vi "f_2_Qgc.vi"(0 "file path (IN)":path, 1 "Project #":string, 2 "Request #":string, 3 "TEST #":string, 5 "error in (no error)":errorcluster, 6 "VGE (-ve)":dbl, 8 "VGE (+ve)":dbl) -> (11 "Di (A)":dbl, 13 "Dt (ns)":dbl, 14 "file path (OUT)":path, 15 "Qgc - Delta Time (us)":dbl, 16 "Di/Dt (A/us)":dbl, 17 "DONE Qgc":bool, 18 "DONE Di/Dt ON":bool, 19 "error out":errorcluster)   [LabVIEW 2020]
uses:
  Global 1.vi
  <vilib>/measure/mamon.llb/Trigger Detection for 1 Channel.vi
  <vilib>/Analysis/NI_AALBase.lvlib
  <vilib>/measure/NI_MAPro.lvlib
panel:
  out "VGE <POINT B>":dbl
  out "Find Major in Histogram":dbl
  out "Histogram":dynamicdata(graph)
  out "Focus graph":waveform(dbl)(graph)
  in  "Decision ?":bool
  out "Dt (us)":dbl
  out "VGE constant point in Median Filter":dbl
  out "VGE <POINT A>":dbl
  out "Cursor c : Channel 2":dbl
  out "Cursor b : Channel 2":dbl
  out "Waveform Graph":waveform(dbl)[](graph)
  out "ON Region":waveform(dbl)[](graph) caption="Qgc"
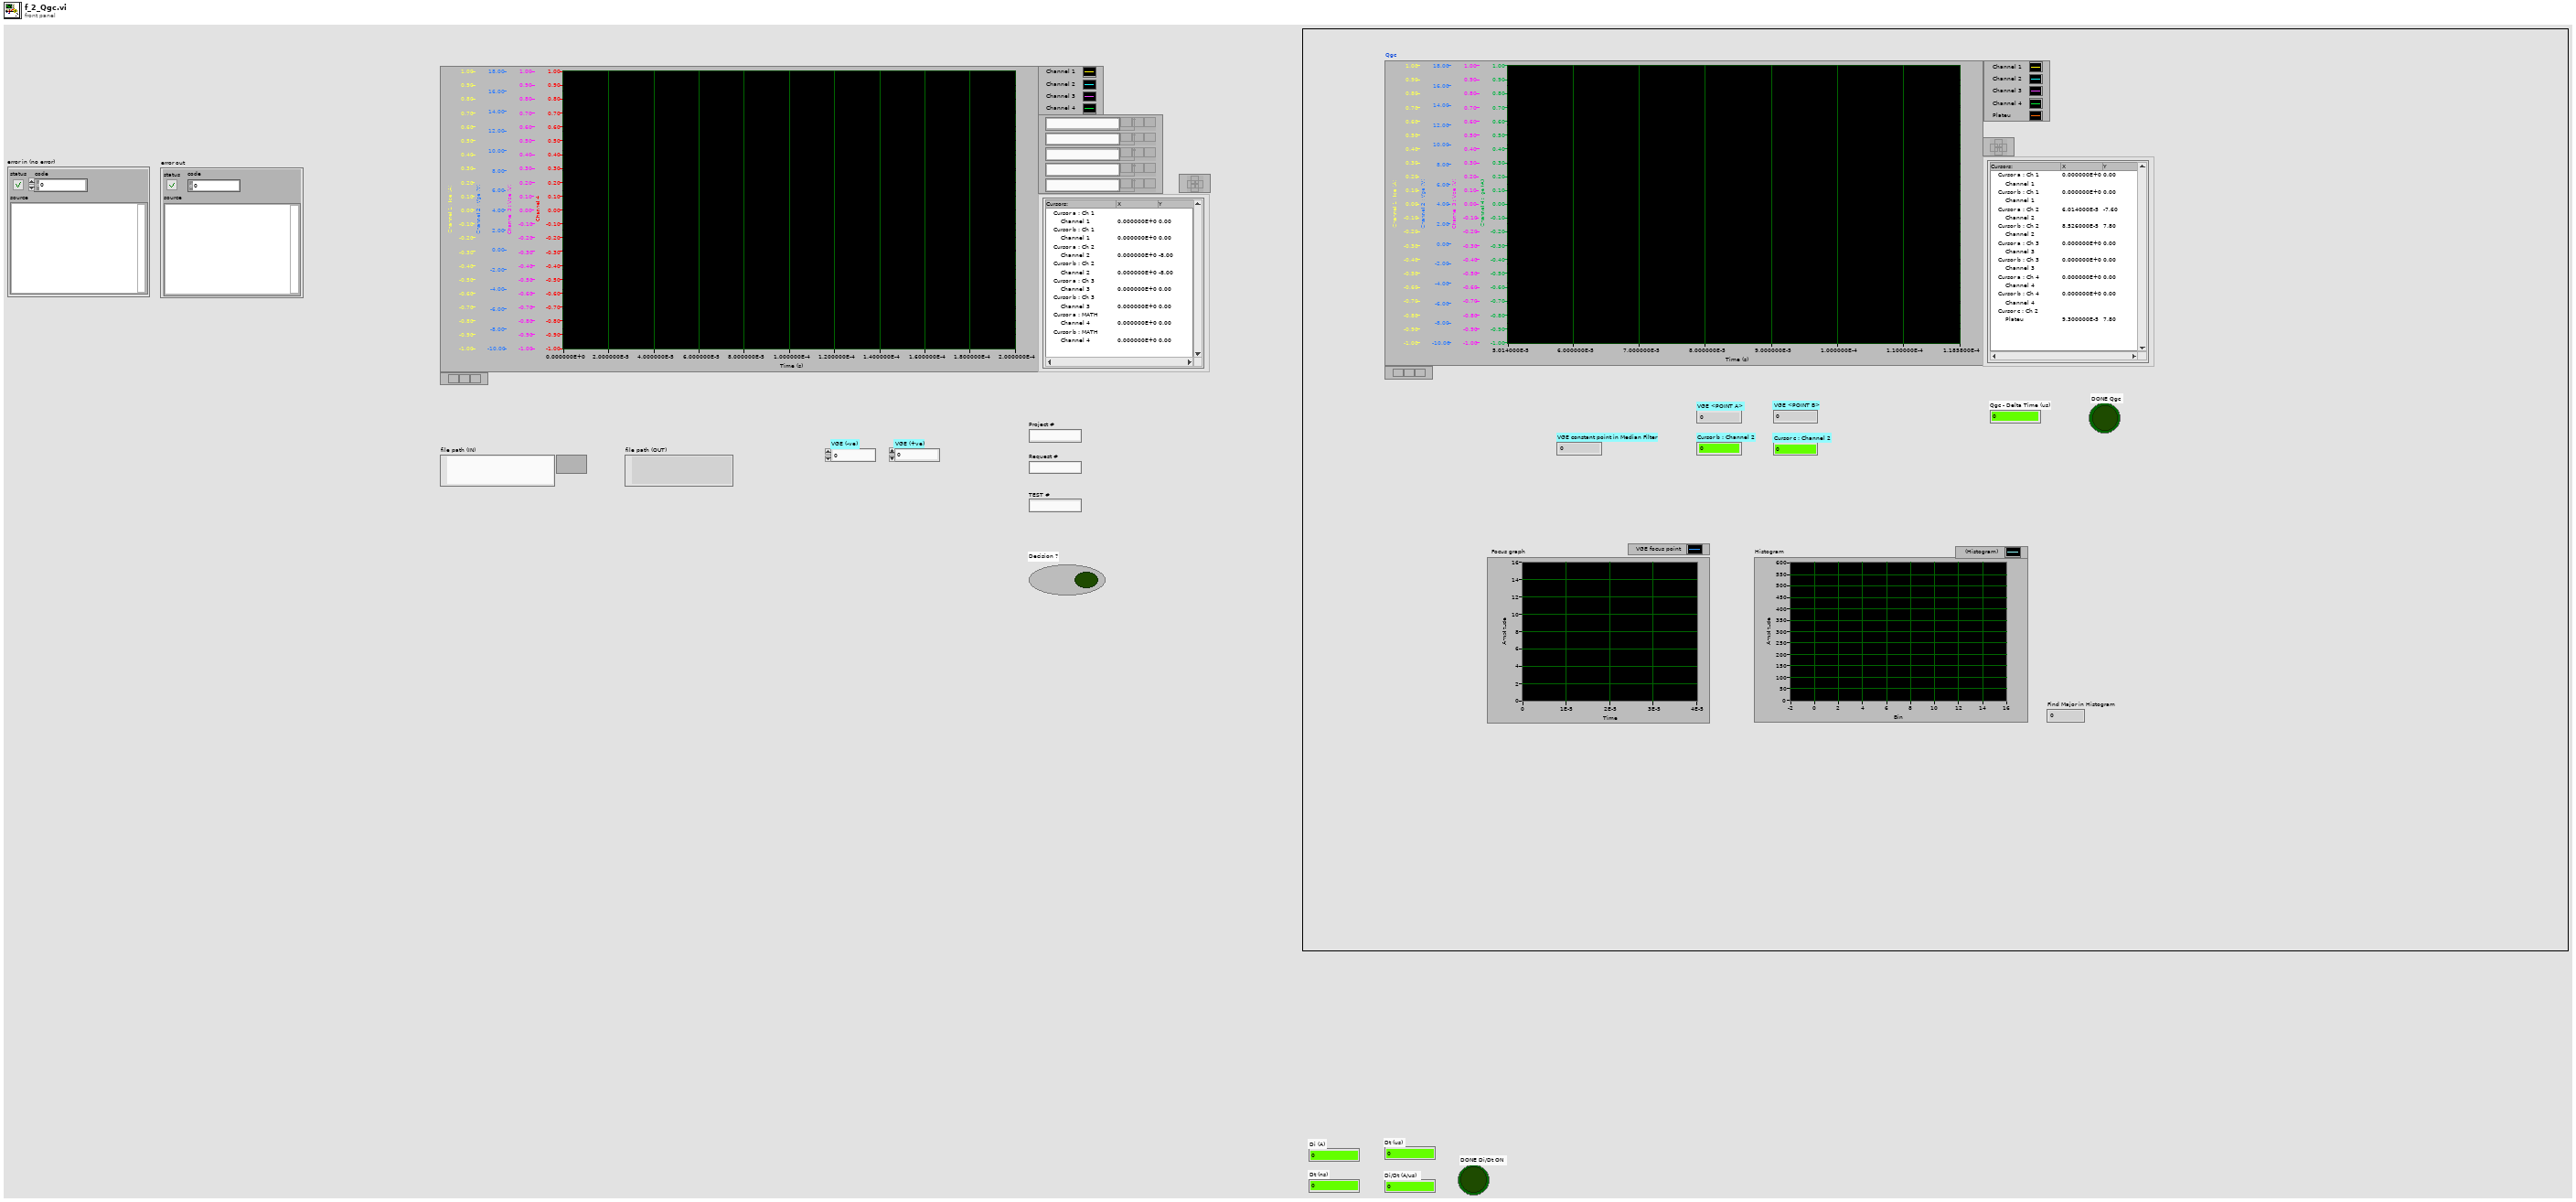
[diagram p1: front panel]
types:
  T1 = enum32{"Invalid", "Standard", "Closed", "Hidden", "Minimized", "Maximized"}
  T2 = typedef "imagedata.ctl" = cluster{"image type":i32, "image depth":i32, "image":u8[], "mask":u8[], "colors":u32[], "Rectangle":cluster{"left":i16, "top":i16, "right":i16, "bottom":i16}}
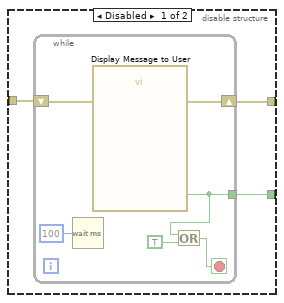
[diagram p2: hidden frame]
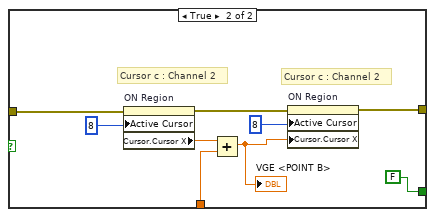
[diagram p9: hidden frame]
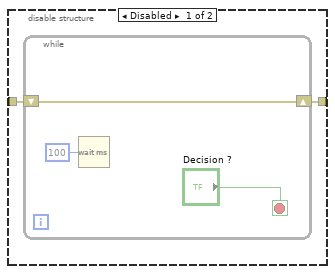
[diagram p11: hidden frame]
diagram:
  w5 = FALSE ("DONE Tdon")
  w1 = 0.0 ("Cursor a : Channel 1")
  w6 = errorcluster {"status"=FALSE, "code"=0, "source"=""} ("error out")
  w7 = waveform(dbl)[] [] ("Waveform Graph")
  n1 = local write "VGE constant point in Median Filter"(w1) -> ()
  n2 = local write "Qgc - Delta Time (us)"(w1) -> ()
  n3 = local write "DONE Qgc"(w5) -> ()
  n4 = local write "Cursor c : Channel 2"(w1) -> ()
  n5 = local write "Cursor b : Channel 2"(w1) -> ()
  n6 = local write "VGE <POINT A>"(w1) -> ()
  n7 = local write "VGE <POINT B>"(w1) -> ()
  n8 = local write "DONE Di/Dt ON"(w5) -> ()
  n9 = local write "Decision ?"(w5) -> ()
  n10 = local write "Di/Dt (A/us)"(w1) -> ()
  n11 = local write "Find Major in Histogram"(0.0 ("Time of Maximum")) -> ()
  n12 = local write "Di (A)"(w1) -> ()
  n13 = local write "Dt (ns)"(w1) -> ()
  n14 = local write "Dt (us)"(w1) -> ()
  n15 = local write "error out"(w6) -> ()
  n16 = local write "error in (no error)"(w6) -> ()
  n17 = local write "Waveform Graph"(w7) -> ()
  n18 = local write "ON Region"(w7) -> ()
  n19 = local write "Histogram"(dynamicdata [] ("Histogram")) -> ()
  n20 = local write "Focus graph"(waveform(dbl) {"t0"=timestamp(0 s since 1904-01-01), "dt"=1.0, "Y"=[]} ("Focus graph")) -> ()
  n21 = flat-sequence {
    tunnel: ["file path (IN)"] -> w13
    tunnel: [w14] -> w12
    tunnel: [w23] -> w11
    tunnel: [w22] -> w10
    tunnel: w13 -> [w25]
    tunnel: w12 -> [w24]
    tunnel: [w402] -> w9
    tunnel: w11 -> [w401]
    tunnel: w10 -> [w400]
    tunnel: [w400] -> w8
    tunnel: w9 -> [w417]
    tunnel: w8 -> [w416]
    frame #0 {
      n22 = control-ref of="This VI"() -> (w19:refnum<vi>)
      n23 = invoke class="VI" method="FP.Open"(reference=w19, error in="error in (no error)", "Activate"=TRUE ("Activate?"), "State"=T1."Maximized") -> (error out=w20:errorcluster)  [unwired: 1 in, 4 out]
      n24 = property class="VI"(reference=w19, error in=w20, "Front Panel.Closeable"=TRUE ("Front Panel Window:Closeable")) -> (error out=w14:errorcluster)  [unwired: 1 out]
    }
    frame #1 {
      n25 = while {
        tunnel: w25 -> [w85]
        shift-right: [w80] -> w23
        shift-left: w24 -> [w84]
        tunnel: [w82] -> w22
        stop <- w79 stop-if-true
        n26 = flat-sequence {
          tunnel: [w113] -> w94
          tunnel: [w114] -> w93
          tunnel: w85 -> [w114]
          tunnel: w84 -> [w113]
          tunnel: w94 -> [w132]
          tunnel: w93 -> [w130]
          tunnel: [w129] -> w75
          tunnel: [w121] -> w74
          tunnel: [w115] -> w73
          tunnel: [w116] -> w72
          tunnel: [w117] -> w71
          tunnel: [w119] -> w70
          tunnel: [w116] -> w46
          tunnel: w75 -> [w173]
          tunnel: [w173] -> w69
          tunnel: w74 -> [w172]
          tunnel: [w172] -> w67
          tunnel: w73 -> [w164]
          tunnel: w72 -> [w171]
          tunnel: w71 -> [w170]
          tunnel: [w170] -> w68
          tunnel: w70 -> [w169]
          tunnel: [w162] -> w66
          tunnel: w46 -> [w161]
          tunnel: [w161] -> w45
          tunnel: [w187] -> w78
          tunnel: w69 -> [w244]
          tunnel: [w244] -> w77
          tunnel: w68 -> [w243]
          tunnel: [w243] -> w76
          tunnel: w67 -> [w200]
          tunnel: w66 -> [w193]
          tunnel: w45 -> [w185]
          tunnel: [w185] -> w44
          tunnel: w78 -> [w258]
          tunnel: [w265] -> w58
          tunnel: w77 -> [w271]
          tunnel: [w271] -> w57
          tunnel: [w264] -> w56
          tunnel: [w245] -> w55
          tunnel: [w259] -> w54
          tunnel: w76 -> [w248]
          tunnel: [w248] -> w53
          tunnel: w44 -> [w247]
          tunnel: [w247] -> w43
          tunnel: w58 -> [w277]
          tunnel: [w284] -> w52
          tunnel: w57 -> [w291]
          tunnel: [w291] -> w51
          tunnel: w56 -> [w290]
          tunnel: [w290] -> w50
          tunnel: w55 -> [w283]
          tunnel: [w283] -> w49
          tunnel: w54 -> [w289]
          tunnel: [w289] -> w48
          tunnel: w53 -> [w288]
          tunnel: [w288] -> w47
          tunnel: w43 -> [w281]
          tunnel: [w281] -> w42
          tunnel: w52 -> [w294]
          tunnel: [w292] -> w41
          tunnel: w51 -> [w299]
          tunnel: [w299] -> w39
          tunnel: w50 -> [w298]
          tunnel: [w298] -> w36
          tunnel: w49 -> [w297]
          tunnel: [w297] -> w34
          tunnel: w48 -> [w296]
          tunnel: [w296] -> w32
          tunnel: w47 -> [w295]
          tunnel: [w295] -> w30
          tunnel: w42 -> [w293]
          tunnel: w41 -> [w331]
          tunnel: [w330] -> w40
          tunnel: w39 -> [w338]
          tunnel: [w338] -> w38
          tunnel: [w329] -> w37
          tunnel: w36 -> [w337]
          tunnel: [w337] -> w35
          tunnel: w34 -> [w336]
          tunnel: [w336] -> w33
          tunnel: w32 -> [w335]
          tunnel: [w335] -> w31
          tunnel: w30 -> [w334]
          tunnel: [w334] -> w29
          tunnel: [w328] -> w26
          tunnel: w40 -> [w344]
          tunnel: w38 -> [w352]
          tunnel: [w352] -> w65
          tunnel: w37 -> [w351]
          tunnel: [w351] -> w64
          tunnel: w35 -> [w350]
          tunnel: [w350] -> w63
          tunnel: w33 -> [w349]
          tunnel: [w349] -> w62
          tunnel: w31 -> [w348]
          tunnel: [w348] -> w61
          tunnel: [w343] -> w60
          tunnel: [w342] -> w59
          tunnel: w29 -> [w340]
          tunnel: [w339] -> w27
          tunnel: w26 -> [w339]
          tunnel: [w356] -> w92
          tunnel: w65 -> [w362]
          tunnel: [w362] -> w91
          tunnel: w64 -> [w361]
          tunnel: [w361] -> w90
          tunnel: w63 -> [w360]
          tunnel: [w360] -> w89
          tunnel: w62 -> [w358]
          tunnel: [w358] -> w88
          tunnel: w61 -> [w359]
          tunnel: w60 -> [w357]
          tunnel: w59 -> [w355]
          tunnel: [w353] -> w28
          tunnel: w27 -> [w353]
          tunnel: w92 -> [w375]
          tunnel: w91 -> [w386]
          tunnel: [w386] -> w87
          tunnel: w90 -> [w381]
          tunnel: w89 -> [w382]
          tunnel: w88 -> [w380]
          tunnel: [w375] -> w86
          tunnel: w28 -> [w373]
          tunnel: w87 -> [w391]
          tunnel: w86 -> [w393]
          tunnel: [w392] -> w81
          tunnel: [w391] -> w82
          frame #0 {
            w110 = waveform(dbl)[] [] ("Waveform Graph")
            w106 = 0.0 ("Cursor a : Channel 1")
            w112 = FALSE ("DONE Tdon")
            n27 = local write "VGE constant point in Median Filter"(w106) -> ()
            n28 = local write "Qgc - Delta Time (us)"(w106) -> ()
            n29 = local write "DONE Qgc"(w112) -> ()
            n30 = local write "Cursor c : Channel 2"(w106) -> ()
            n31 = local write "Cursor b : Channel 2"(w106) -> ()
            n32 = local write "VGE <POINT B>"(w106) -> ()
            n33 = local write "DONE Di/Dt ON"(w112) -> ()
            n34 = local write "Decision ?"(w112) -> ()
            n35 = local write "Di (A)"(w106) -> ()
            n36 = local write "Dt (ns)"(w106) -> ()
            n37 = local write "Dt (us)"(w106) -> ()
            n38 = local write "Di/Dt (A/us)"(w106) -> ()
            n39 = local write "VGE <POINT A>"(w106) -> ()
            n40 = Wait (ms)(milliseconds to wait=u32 200) -> ()  [unwired: 1 out]
            n41 = local write "Find Major in Histogram"(0.0 ("Time of Maximum")) -> ()
            n42 = local write "Histogram"(dynamicdata [] ("Histogram")) -> ()
            n43 = local write "ON Region"(w110) -> ()
            n44 = local write "Waveform Graph"(w110) -> ()
            n45 = local write "Focus graph"(waveform(dbl) {"t0"=timestamp(0 s since 1904-01-01), "dt"=1.0, "Y"=[]} ("Focus graph")) -> ()
          }
          frame #1 {
            w121 = 0.0 ("number")
            # "Channel 2"
            # "Channel 4"
            # "t0"
            # "Channel 1"
            # "Channel 3"
            # "dt"
            # "Ch1"
            n46 = call "3_ReadDatatoWaveform.vi"("file path (IN)"=w130, "error in (no error)"=w132) -> ("Ch 1 Data"=w128:dbl[], "Ch 2 Data"=w123:dbl[], "file path (OUT)"=w129:path, "Waveform Graph"=→"Waveform Graph":waveform(dbl)[], "Ch 3 Data"=w127:dbl[], "Ch 4 Data"=w125:dbl[], "dt"=w116:dbl, "error out"=w131:errorcluster)  [unwired: 5 in, 1 out]
            n47 = To Time Stamp(1:w121) -> (0:w124:timestamp)
            n48 = disable-structure shown="Enabled" {
              disable-tunnel: w124 -> [w148 _]
              disable-tunnel: w116 -> [w147 _]
              disable-tunnel: w123 -> [w146 _]
              disable-tunnel: [w145 _] -> w118
              frame Enabled {
                # "Channel 2"
                n49 = Bundle By Name("Y"=w146, "dt"=w147, "t0"=w148) -> (w145:waveform(dbl))  [unwired: 1 in]
              }
              frame Disabled {
              }
            }
            n50 = disable-structure shown="Enabled" {
              disable-tunnel: w124 -> [w160 _]
              disable-tunnel: w116 -> [w159 _]
              disable-tunnel: w127 -> [w158 _]
              disable-tunnel: [w157 _] -> w133
              frame Enabled {
                # "Channel 3"
                n51 = Bundle By Name("Y"=w158, "dt"=w159, "t0"=w160) -> (w157:waveform(dbl))  [unwired: 1 in]
              }
              frame Disabled {
              }
            }
            n52 = disable-structure shown="Enabled" {
              disable-tunnel: w124 -> [w152 _]
              disable-tunnel: w116 -> [w151 _]
              disable-tunnel: w125 -> [w150 _]
              disable-tunnel: [w149 _] -> w120
              frame Enabled {
                # "Channel 4"
                n53 = Bundle By Name("Y"=w150, "dt"=w151, "t0"=w152) -> (w149:waveform(dbl))  [unwired: 1 in]
              }
              frame Disabled {
              }
            }
            n54 = disable-structure shown="Enabled" {
              disable-tunnel: w124 -> [w156 _]
              disable-tunnel: w116 -> [w155 _]
              disable-tunnel: w128 -> [w154 _]
              disable-tunnel: [w153 _] -> w134
              frame Enabled {
                # "Channel 1"
                n55 = Bundle By Name("Y"=w154, "dt"=w155, "t0"=w156) -> (w153:waveform(dbl))  [unwired: 1 in]
              }
              frame Disabled {
              }
            }
            n56 = property on="Waveform Graph" class="WFGraph (strict)"(error in=w131, "XScale.Offset"=w121) -> (error out=w115:errorcluster)  [unwired: 1 in, 1 out]
            n57 = disable-structure shown="Enabled" {
              disable-tunnel: w118 -> [w143 _]
              disable-tunnel: [w142 _] -> w117
              disable-tunnel: [w141 _] -> w119
              disable-tunnel: w116 -> [w140 _]
              frame Enabled {
                # "OG = 30"
                # "Median"
                n58 = global read "Global 1.vi" "Median Filter Rank"() -> (w139:i32)
                n59 = Unbundle By Name(w143) -> ("Y"=w144:dbl[])
                n60 = call <vilib>:"Median Filter.vi"("right rank"=w139, "left rank"=w139, "X"=w144) -> ("Filtered X"=w141:dbl[])  [unwired: 7 in, 1 out]
                n61 = Bundle By Name("Y"=w141, "dt"=w140) -> (w142:waveform(dbl))  [unwired: 1 in]
              }
              frame Disabled {
              }
            }
            n62 = Build Array(w134, w118, w133, w120, w117) -> (→"ON Region":waveform(dbl)[])
            n63 = Wait (ms)(milliseconds to wait=u32 200) -> ()  [unwired: 1 out]
            n64 = call <vilib>:"Beep.vi"("use system alert? (T)"=FALSE, "duration (msec)"=u32 200, "frequency (Hz)"=u32 2000) -> ()  [unwired: 9 in]
          }
          frame #2 {
            n65 = disable-structure shown="Enabled" {
              disable-tunnel: w171 -> [_ w179]
              disable-tunnel: w169 -> [_ w175]
              disable-tunnel: [_ w174] -> w167
              frame Disabled {
              }
              frame Enabled {
                # "Remains"
                # "Find (+ve)"
                # "Find 0"
                n66 = Search 1D Array(1D array=w175, element=0.0, start index (0)=0) -> (index of element=w180:i32)
                n67 = Split 1D Array(array=w175, index=w180) -> (second subarray=w183:dbl[])  [unwired: 1 out]
                n68 = Search 1D Array(1D array=w183, element="VGE (+ve)", start index (0)=0) -> (index of element=w182:i32)
                n69 = Split 1D Array(array=w183, index=w182) -> (first subarray=w184:dbl[])  [unwired: 1 out]
                n70 = Bundle By Name("Y"=w184, "dt"=w179) -> (w174:waveform(dbl))  [unwired: 1 in]
                "Focus graph" <- w174
              }
            }
            n71 = Wait (ms)(milliseconds to wait=u32 200) -> ()  [unwired: 1 out]
            n72 = call "Create Histogram"("error in (no error)"=w164, "Signal"=w167) -> ("error out"=w163:errorcluster, "Histogram"=w166:dynamicdata)  [unwired: 8 in]
            "Histogram" <- w166
            n73 = call "Statistics"("Signals"=w166, "error in (no error)"=w163) -> ("Time of Maximum"=→"Find Major in Histogram":dynamicdata, "error out"=w162:errorcluster)  [unwired: 24 in]
          }
          frame #3 {
            n74 = property on="ON Region" class="WFGraph (strict)"(error in=w193) -> (error out=w201:errorcluster, "Width"=w202:u32)  [unwired: 1 in, 1 out]
            n75 = property on="ON Region" class="WFGraph (strict)"(error in=w201, "Caption.Justify"=enum16{"Left", "Center", "Right"}."Left" ("Caption.Justification"), "Caption.Width"=w202, "Caption.FontBold"=TRUE ("Caption.Font:Bold"), "Caption.FontColor"=u32 16860 ("Caption.Font:Color"), "Caption.FontSize"=u32 24 ("Caption.Font:Size"), "Caption.Text"="Qgc") -> (error out=w203:errorcluster)  [unwired: 1 in, 1 out]
            n76 = Wait (ms)(milliseconds to wait=u32 200) -> ()  [unwired: 1 out]
            n77 = property on="ON Region" class="WFGraph (strict)"(error in=w203, "XScale.Offset"=w200) -> (error out=w194:errorcluster)  [unwired: 1 in, 1 out]
            n78 = property on="ON Region" class="WFGraph (strict)"(error in=w194, "Active Cursor"=u32 0, "Cursor.Cursor X"=0.0 ("Cursor.Cursor Position:Cursor X"), "Cursor.Cursor Y"=0.0 ("Cursor.Cursor Position:Cursor Y"), "Cursor.Visible"=FALSE) -> (error out=w236:errorcluster)  [unwired: 1 in, 1 out]
            n79 = property on="ON Region" class="WFGraph (strict)"(error in=w236, "Active Cursor"=u32 1, "Cursor.Cursor X"=0.0 ("Cursor.Cursor Position:Cursor X"), "Cursor.Cursor Y"=0.0 ("Cursor.Cursor Position:Cursor Y"), "Cursor.Visible"=FALSE) -> (error out=w237:errorcluster)  [unwired: 1 in, 1 out]
            n80 = property on="ON Region" class="WFGraph (strict)"(error in=w237, "Active Cursor"=u32 2, "Cursor.Cursor X"=0.0 ("Cursor.Cursor Position:Cursor X"), "Cursor.Cursor Y"=0.0 ("Cursor.Cursor Position:Cursor Y"), "Cursor.Visible"=FALSE) -> (error out=w238:errorcluster)  [unwired: 1 in, 1 out]
            n81 = property on="ON Region" class="WFGraph (strict)"(error in=w238, "Active Cursor"=u32 3, "Cursor.Cursor X"=0.0 ("Cursor.Cursor Position:Cursor X"), "Cursor.Cursor Y"=0.0 ("Cursor.Cursor Position:Cursor Y"), "Cursor.Visible"=FALSE) -> (error out=w239:errorcluster)  [unwired: 1 in, 1 out]
            n82 = property on="ON Region" class="WFGraph (strict)"(error in=w239, "Active Cursor"=u32 4, "Cursor.Cursor X"=0.0 ("Cursor.Cursor Position:Cursor X"), "Cursor.Cursor Y"=0.0 ("Cursor.Cursor Position:Cursor Y"), "Cursor.Visible"=FALSE) -> (error out=w240:errorcluster)  [unwired: 1 in, 1 out]
            n83 = property on="ON Region" class="WFGraph (strict)"(error in=w240, "Active Cursor"=u32 5, "Cursor.Cursor X"=0.0 ("Cursor.Cursor Position:Cursor X"), "Cursor.Cursor Y"=0.0 ("Cursor.Cursor Position:Cursor Y"), "Cursor.Visible"=FALSE) -> (error out=w241:errorcluster)  [unwired: 1 in, 1 out]
            n84 = property on="ON Region" class="WFGraph (strict)"(error in=w241, "Active Cursor"=u32 6, "Cursor.Cursor X"=0.0 ("Cursor.Cursor Position:Cursor X"), "Cursor.Cursor Y"=0.0 ("Cursor.Cursor Position:Cursor Y"), "Cursor.Visible"=FALSE) -> (error out=w242:errorcluster)  [unwired: 1 in, 1 out]
            n85 = property on="ON Region" class="WFGraph (strict)"(error in=w242, "Active Cursor"=u32 7, "Cursor.Cursor X"=0.0 ("Cursor.Cursor Position:Cursor X"), "Cursor.Cursor Y"=0.0 ("Cursor.Cursor Position:Cursor Y"), "Cursor.Visible"=FALSE) -> (error out=w188:errorcluster)  [unwired: 1 in, 1 out]
            n86 = property on="ON Region" class="WFGraph (strict)"(error in=w188, "Active Cursor"=u32 8, "Cursor.Cursor X"=0.0 ("Cursor.Cursor Position:Cursor X"), "Cursor.Cursor Y"=0.0 ("Cursor.Cursor Position:Cursor Y"), "Cursor.Visible"=FALSE) -> (error out=w187:errorcluster)  [unwired: 1 in, 1 out]
          }
          frame #4 {
            w255 = u16 1 items=["Falling Edge", "Rising Edge"] ("trigger slope")
            w256 = u16 1 items=["Index", "Time"] ("location mode")
            w260 = u16 1 items=["Falling Edge", "Rising Edge"] ("trigger slope")
            w261 = u16 1 items=["Index", "Time"] ("location mode")
            # "Cursor a : Channel 2"
            # "Cursor b : Channel 2"
            # "Cursor b : Channel 2"
            # "Cursor b : Channel 2"
            # "Cursor b : Channel 2"
            # "Cursor a : Channel 2"
            # "End Time 1st Cursor"
            # "End Time 2nd Cursor"
            # "1st PARAMETER : VGE (-ve)"
            # "Channel 2"
            # "2nd PARAMETER : VGE constant point"
            # "Channel 2"
            n87 = Add(x="VGE (-ve)", y=0.3) -> (x+y=w251:dbl)
            n88 = call-poly <vilib>:"Basic Level Trigger Detection.vi"("signal in"=w248, "level"=w251, "location mode"=w261, "error in (no error)"=w258, "trigger slope"=w260) -> ("trigger location"=w259:dbl, "error out"=w257:errorcluster)  [unwired: 8 in, 1 out]
            n89 = property on="ON Region" class="WFGraph (strict)"(error in=w257, "Active Cursor"=u32 2, "Cursor.Cursor X"=w259, "Cursor.Visible"=TRUE, "Cursor.Cursor Name Visible"=TRUE) -> (error out=w246:errorcluster)  [unwired: 1 in, 1 out]
            n90 = local read "Find Major in Histogram"() -> (w253:dbl)
            "VGE constant point in Median Filter" <- w253
            n91 = call-poly <vilib>:"Basic Level Trigger Detection.vi"("signal in"=w248, "level"=w253, "location mode"=w256, "error in (no error)"=w246, "trigger slope"=w255) -> ("trigger location"=w245:dbl, "error out"=w254:errorcluster)  [unwired: 8 in, 1 out]
            "VGE <POINT A>" <- w245
            n92 = Wait (ms)(milliseconds to wait=u32 200) -> ()  [unwired: 1 out]
            n93 = property on="ON Region" class="WFGraph (strict)"(error in=w254, "Active Cursor"=u32 3, "Cursor.Cursor X"=w245, "Cursor.Visible"=TRUE, "Cursor.Cursor Name Visible"=TRUE) -> (error out=w266:errorcluster)  [unwired: 1 in, 1 out]
            n94 = call <vilib>:"Beep.vi"("use system alert? (T)"=FALSE, "duration (msec)"=u32 200, "frequency (Hz)"=u32 2000) -> ()  [unwired: 9 in]
            n95 = property on="ON Region" class="WFGraph (strict)"(error in=w266, "Active Cursor"=u32 3) -> (error out=w265:errorcluster, "Cursor.Cursor Y"=w264:dbl)  [unwired: 1 in, 1 out]
            "Cursor b : Channel 2" <- w264
          }
          frame #5 {
            # "Cursor a : Channel 2"
            # "Cursor c : Channel 2"
            n96 = Wait (ms)(milliseconds to wait=u32 200) -> ()  [unwired: 1 out]
            n97 = property on="ON Region" class="WFGraph (strict)"(error in=w277, "Active Cursor"=u32 2, "Cursor.Visible"=FALSE, "Cursor.Cursor Name Visible"=FALSE) -> (error out=w276:errorcluster)  [unwired: 1 in, 1 out]
            n98 = property on="ON Region" class="WFGraph (strict)"(error in=w276, "Active Cursor"=u32 8, "Cursor.Cursor X"=w283, "Cursor.Visible"=TRUE, "Cursor.Cursor Name Visible"=TRUE) -> (error out=w284:errorcluster)  [unwired: 1 in, 1 out]
          }
          frame #6 {
            n99 = while {
              tunnel: w293 -> [w304]
              shift-right: [w300] -> w292
              shift-left: w294 -> [w306]
              stop <- w302 stop-if-true
              # "Cursor c : Channel 2"
              n100 = local read "Cursor b : Channel 2"() -> (w307:dbl)
              n101 = property on="ON Region" class="WFGraph (strict)"(error in=w306, "Active Cursor"=u32 8) -> (error out=w301:errorcluster, "Cursor.Cursor Y"=w308:dbl)  [unwired: 1 in, 1 out]
              n102 = Equal?(x=w308, y=w307) -> (x = y?=w305:bool)
              n103 = case shown="False" w305 {
                tunnel: w304 -> [w311 w323]
                tunnel: [TRUE FALSE] -> w302
                tunnel: w301 -> [w313 w321]
                tunnel: [w312 w320] -> w300
                frame False {
                  # "Cursor c : Channel 2"
                  # "Cursor c : Channel 2"
                  n104 = property on="ON Region" class="WFGraph (strict)"(error in=w313, "Active Cursor"=u32 8) -> (error out=w316:errorcluster, "Cursor.Cursor X"=w317:dbl)  [unwired: 1 in, 1 out]
                  n105 = Subtract(x=w317, y=w311) -> (x-y=w310:dbl)
                  n106 = local write "VGE <POINT B>"(w310) -> ()
                  n107 = property on="ON Region" class="WFGraph (strict)"(error in=w316, "Active Cursor"=u32 8, "Cursor.Cursor X"=w310) -> (error out=w312:errorcluster)  [unwired: 1 in, 1 out]
                }
                frame True {
                  # "Cursor c : Channel 2"
                  # "Cursor c : Channel 2"
                  n108 = property on="ON Region" class="WFGraph (strict)"(error in=w321, "Active Cursor"=u32 8) -> (error out=w324:errorcluster, "Cursor.Cursor X"=w325:dbl)  [unwired: 1 in, 1 out]
                  n109 = Add(x=w325, y=w323) -> (x+y=w319:dbl)
                  "VGE <POINT B>" <- w319
                  n110 = property on="ON Region" class="WFGraph (strict)"(error in=w324, "Active Cursor"=u32 8, "Cursor.Cursor X"=w319) -> (error out=w320:errorcluster)  [unwired: 1 in, 1 out]
                }
              }
              n111 = Wait (ms)(milliseconds to wait=u32 1) -> ()  [unwired: 1 out]
            }
          }
          frame #7 {
            # "Cursor c : Channel 2"
            n112 = property on="ON Region" class="WFGraph (strict)"(error in=w331, "Active Cursor"=u32 8) -> (error out=w330:errorcluster, "Cursor.Cursor Y"=w329:dbl, "Cursor.Cursor X"=w328:dbl)  [unwired: 1 in, 1 out]
            "Cursor c : Channel 2" <- w329
            n113 = Wait (ms)(milliseconds to wait=u32 200) -> ()  [unwired: 1 out]
          }
          frame #8 {
            w346 = u16 1 items=["Falling Edge", "Rising Edge"] ("trigger slope")
            w345 = u16 1 items=["Index", "Time"] ("location mode")
            # "VGE +ve"
            # "Channel 2"
            n114 = local read "VGE (+ve)"() -> (w347:dbl)
            n115 = Wait (ms)(milliseconds to wait=u32 200) -> ()  [unwired: 1 out]
            n116 = call-poly <vilib>:"Basic Level Trigger Detection.vi"("signal in"=w340, "level"=w347, "location mode"=w345, "error in (no error)"=w344, "trigger slope"=w346) -> ("trigger location"=w342:dbl, "error out"=w343:errorcluster)  [unwired: 8 in, 1 out]
          }
          frame #9 {
            n117 = Wait (ms)(milliseconds to wait=u32 200) -> ()  [unwired: 1 out]
            n118 = disable-structure shown="Enabled" {
              disable-tunnel: w357 -> [w370 w371]
              disable-tunnel: [w369 w371] -> w356
              disable-tunnel: w359 -> [w364 _]
              disable-tunnel: w355 -> [w363 _]
              frame Enabled {
                # "2nd Cursor"
                # "1st Cursor"
                n119 = Subtract(x=w364, y=1e-05) -> (x-y=w365:dbl)
                n120 = Add(x=w363, y=1e-05) -> (x+y=w366:dbl)
                n121 = property on="ON Region" class="WFGraph (strict)"(error in=w370, "XScale.Minimum"=w365, "XScale.Maximum"=w366) -> (error out=w369:errorcluster)  [unwired: 1 in, 1 out]
              }
              frame Disabled {
              }
            }
          }
          frame #10 {
            # "us"
            # "ns"
            n122 = Subtract(x=w382, y=w381) -> (x-y=w378:dbl)
            n123 = Subtract(x=w380, y=w373) -> (x-y=w379:dbl)
            n124 = Absolute Value(x=w378) -> (abs(x)=w377:dbl)
            "Di (A)" <- w377
            n125 = Absolute Value(x=w379) -> (abs(x)=w376:dbl)
            n126 = Multiply(x=w376, y=1000000000.0) -> (x*y=→"Dt (ns)":dbl)
            n127 = Multiply(x=w376, y=1000000.0) -> (x*y=w372:dbl)
            "Qgc - Delta Time (us)" <- w372
            "Dt (us)" <- w372
            n128 = call <vilib>:"Beep.vi"("use system alert? (T)"=FALSE, "duration (msec)"=u32 200, "frequency (Hz)"=u32 2000) -> ()  [unwired: 9 in]
            n129 = Divide(x=w377, y=w372) -> (x/y=→"Di/Dt (A/us)":dbl)
            n130 = Wait (ms)(milliseconds to wait=u32 200) -> ()  [unwired: 1 out]
          }
          frame #11 {
            n131 = disable-structure shown="Enabled" {
              disable-tunnel: w393 -> [w395 w399]
              disable-tunnel: [w394 w399] -> w392
              frame Disabled {
                n132 = while {
                  shift-right: [w396] -> w394
                  shift-left: w395 -> [w396]
                  stop <- "Decision ?" stop-if-true
                  n133 = Wait (ms)(milliseconds to wait=u32 100) -> ()  [unwired: 1 out]
                }
              }
              frame Enabled {
              }
            }
          }
        }
        n134 = disable-structure shown="Enabled" {
          disable-tunnel: w81 -> [w97 w104]
          disable-tunnel: [w96 w104] -> w80
          disable-tunnel: [w95 TRUE ("NO")] -> w79
          frame Disabled {
            n135 = while {
              tunnel: [w99] -> w95
              shift-right: [w102] -> w96
              shift-left: w97 -> [w103]
              stop <- w101 stop-if-true
              n136 = Wait (ms)(milliseconds to wait=u32 100) -> ()  [unwired: 1 out]
              n137 = call "Display Message to User"("error in (no error)"=w103) -> ("error out"=w102:errorcluster, "NO"=w99:bool)  [unwired: 9 in]
              n138 = Or(x=w99, y=TRUE) -> (x .or. y?=w101:bool)
            }
          }
          frame Enabled {
          }
        }
        n139 = Wait (ms)(milliseconds to wait=u32 100) -> ()  [unwired: 1 out]
      }
    }
    frame #2 {
      w405 = "_"
      n140 = invoke on="ON Region" class="WFGraph (strict)" method="Get Image"(error in=w401) -> (error out=w409:errorcluster, "image data"=w412:T2)  [unwired: 5 in, 4 out]
      n141 = Concatenate Strings("C:\\GateCharge_Project\\GateCharge_Image\\" ("string"), "Project #", w405, "Request #", w405, "TEST #", w405, "Qgc" ("string"), ".png" ("string")) -> (w413:string)
      n142 = String To Path(string=w413) -> (path=w411:path)
      n143 = call <vilib>:"Write PNG File.vi"("error in (no error)"=w409, "image data"=w412, "path to PNG file"=w411) -> ("error out"=w402:errorcluster)  [unwired: 7 in, 1 out]
      "DONE Qgc" <- TRUE ("DONE Tdon")
      "DONE Di/Dt ON" <- TRUE ("DONE Di/Dt ON")
    }
    frame #3 {
      n144 = disable-structure shown="Enabled" {
        disable-tunnel: w417 -> [w418 _]
        frame Enabled {
          n145 = control-ref of="This VI"() -> (w419:refnum<vi>)
          n146 = invoke class="VI" method="FP.Close"(reference=w419, error in=w418) -> ()  [unwired: 1 in, 3 out]
        }
        frame Disabled {
        }
      }
      "error out" <- w417
      "file path (OUT)" <- w416
    }
  }
